vi "runCtrChgAfterTime.vi"(1 "init(ticks)":u32, 2 "timeDif(ticks)":u32) -> (0 "change":bool)   [LabVIEW 2014]
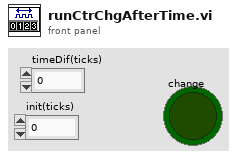
[diagram p1: front panel]
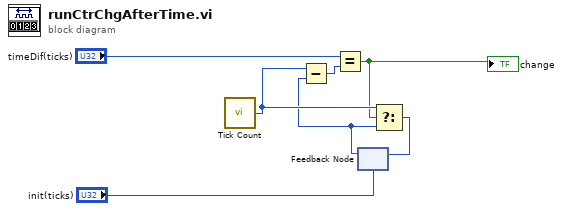
[diagram p0: block diagram]
diagram:
  n1 = call "Tick Count"() -> ("Tick Count(Ticks)"=w7:u32)
  n2 = feedback #1("init(ticks)") -> (w5:u32)
  n3 = Subtract(x=w7, y=w5) -> (x-y=w4:u32)
  n4 = Equal?(x="timeDif(ticks)", y=w4) -> (x = y?=w3:bool)
  "change" <- w3
  n5 = Select(t=w7, s=w3, f=w5) -> (s? t:f=w6:u32)
  n6 = feedback-in #1(w6) -> ()
